vi "Get Operators.vi"(11 "Expression":string) -> (3 "Operators":string[](array[string]))   [LabVIEW 2018]
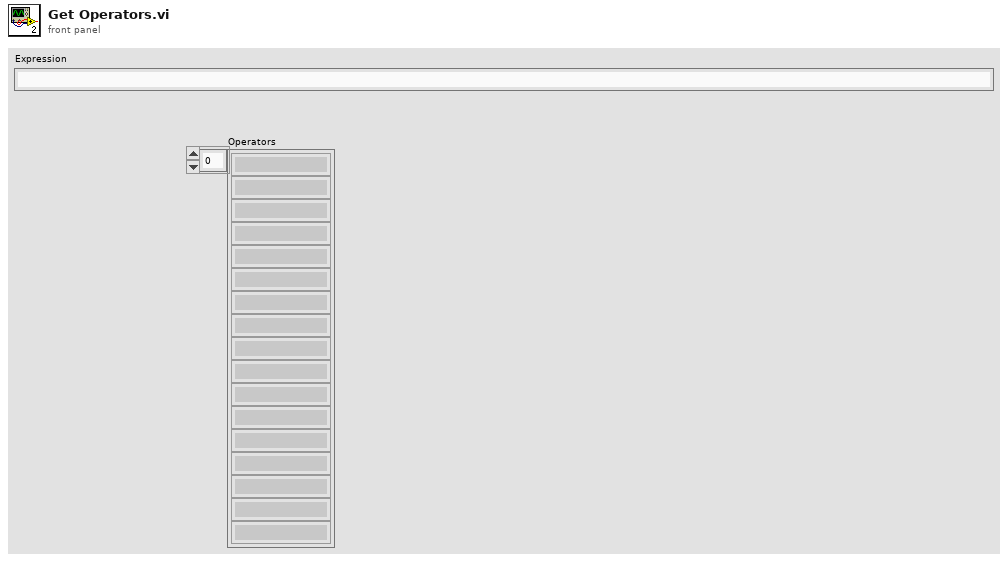
[diagram p1: front panel]
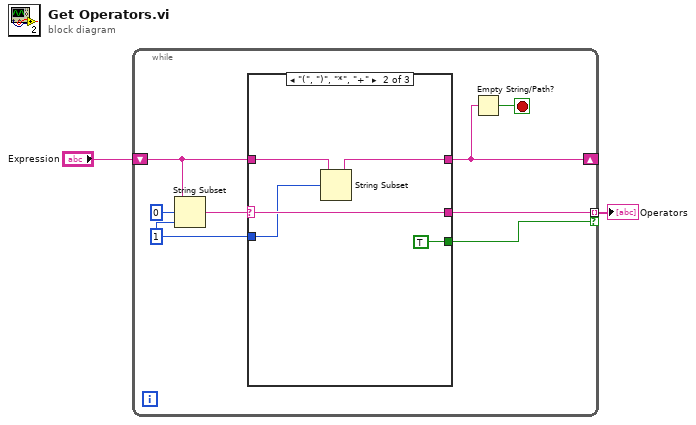
[diagram p0: block diagram]
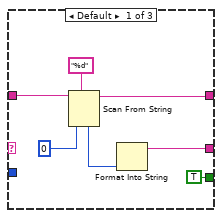
[diagram p2: hidden frame]
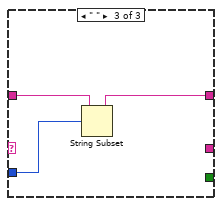
[diagram p3: hidden frame]
diagram:
  n1 = while {
    shift-right: [w5] -> _
    shift-left: "Expression" -> [w7]
    tunnel: [w8] -> w1 mode=indexing if=w3
    stop <- w4 stop-if-true
    w6 = 1
    n2 = String Subset(string=w7, offset (0)=0, length (rest)=w6) -> (substring=w9:string)
    n3 = case shown="\"(\", \")\", \"*\", \"+\"" w9 {
      selector: w9 -> [_ w22 _]
      tunnel: [w12 w22 _] -> w8
      tunnel: w7 -> [w17 w21 w25]
      tunnel: [w16 w19 w23] -> w5
      tunnel: w6 -> [_ w20 w24]
      tunnel: [TRUE TRUE _] -> w3
      frame Default {
        n4 = Scan From String(format string="%d", input string=w17, default 1=0) -> (remaining string=w16:string, output 1=w13:i32)  [unwired: 2 in, 2 out]
        n5 = Format Into String(w13) -> (resulting string=w12:string)  [unwired: 3 in, 1 out]
      }
      frame "(", ")", "*", "+" {
        n6 = String Subset(string=w21, offset (0)=w20) -> (substring=w19:string)  [unwired: 1 in]
      }
      frame " " {
        n7 = String Subset(string=w25, offset (0)=w24) -> (substring=w23:string)  [unwired: 1 in]
      }
    }
    n8 = Empty String/Path?(string/path=w5) -> (empty?=w4:bool)
  }
  "Operators" <- w1
